vi "FunctionGenerator_New.vi"(11 "X Y Pairs":T1[](array[typedef]) {"Y" format="%_7f"; "X" format="%_7f"}) -> (3 "FUNCTION_GENERATOR":T2)   [LabVIEW 2019, in "Trajectory_Library.lvlib"]
doc: "Create a new Funtion Generator. Function Generators (Interpolating Tree Maps) are used to get values at points that are not defined by making a guess from points that are defined. This uses linear interpolation.\n\nInputs:\n - X Y Pairs -- (Optional) Array of pairs of X and Y values used to define this function generator. Additional X Y pairs can be added later. \n\nOutputs:\n - Function Generator -- Created data structure"
uses:
  Trajectory_Library.lvlib
  TypeDef/FUNCTION_GENERATOR.ctl
  X_Y_PAIR.ctl
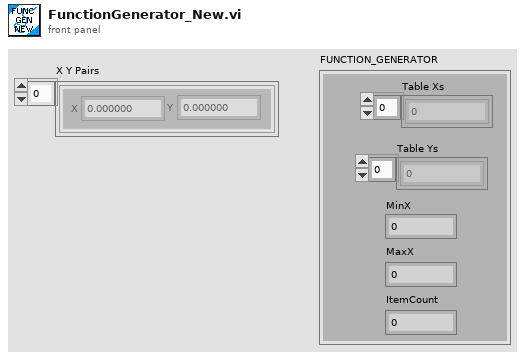
[diagram p1: front panel]
types:
  T1 = typedef "Trajectory_Library.lvlib/X_Y_PAIR.ctl" = cluster{"X":dbl, "Y":dbl}
  T2 = typedef "Trajectory_Library.lvlib/FUNCTION_GENERATOR.ctl" = cluster{"Table Xs":dbl[], "Table Ys":dbl[], "MinX":dbl, "MaxX":dbl, "ItemCount":i32}
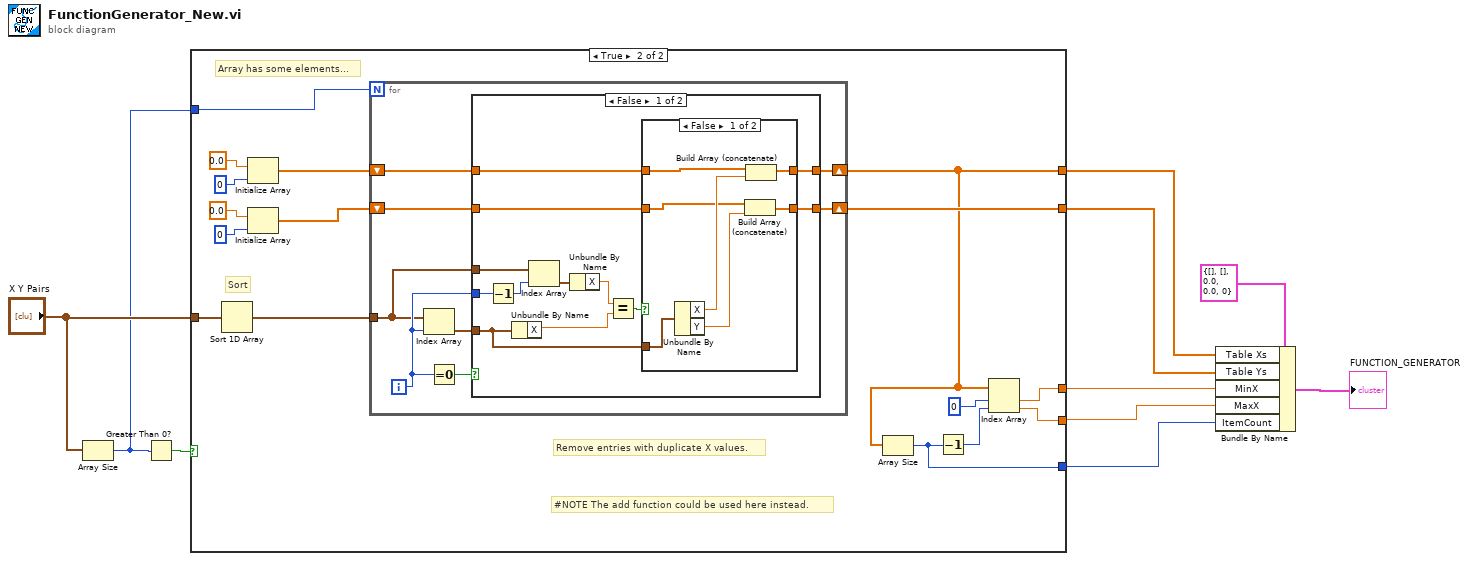
[diagram p0: block diagram]
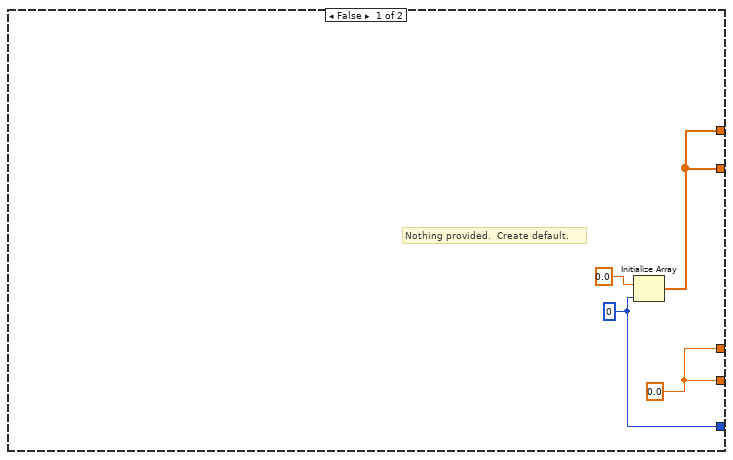
[diagram p2: hidden frame]
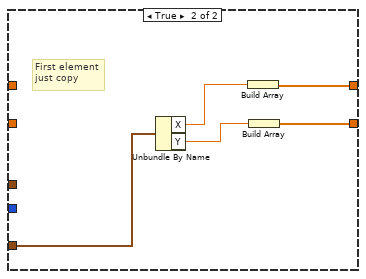
[diagram p4: hidden frame]
diagram:
  n1 = Array Size(array="X Y Pairs") -> (size(s)=w6:i32)
  n2 = Greater Than 0?(x=w6) -> (x > 0?=w8:bool)
  n3 = case shown="True" w8 {
    tunnel: "X Y Pairs" -> [_ w30]
    tunnel: w6 -> [_ w27]
    tunnel: [w13 w17] -> w5
    tunnel: [w13 w18] -> w4
    tunnel: [w12 w16] -> w3
    tunnel: [w12 w15] -> w2
    tunnel: [w11 w24] -> w1
    frame False {
      w12 = 0.0 ("X")
      w11 = 0 ("dimension size")
      # "Nothing provided.  Create default."
      n4 = Initialize Array(0.0 ("element"), w11) -> (w13:dbl[])
    }
    frame True {
      # "#NOTE The add function could be used here instead."
      # "Remove entries with duplicate X values."
      # "Sort"
      # "Array has some elements..."
      n5 = Sort 1D Array(array=w30) -> (sorted array=w26:T1[])
      n6 = Initialize Array(0.0, 0 ("dimension size")) -> (w20:dbl[])
      n7 = Initialize Array(0.0, 0 ("dimension size")) -> (w19:dbl[])
      n8 = for {
        N: w27 -> [_]
        tunnel: w26 -> [w35]
        shift-right: [w34] -> w17
        shift-left: w20 -> [w32]
        shift-right: [w33] -> w18
        shift-left: w19 -> [w31]
        i -> [w36]
        n9 = Index Array(array=w35, index=w36) -> (element=w37:T1)
        n10 = Equal To 0?(x=w36) -> (x = 0?=w38:bool)
        n11 = case shown="False" w38 {
          tunnel: w37 -> [w43 w64]
          tunnel: w36 -> [w49 _]
          tunnel: w35 -> [w48 _]
          tunnel: [w42 w63] -> w34
          tunnel: [w41 w62] -> w33
          tunnel: w32 -> [w40 _]
          tunnel: w31 -> [w39 _]
          frame False {
            n12 = Decrement(x=w49) -> (x-1=w50:i32)
            n13 = Unbundle By Name(w43) -> ("X"=w45:dbl)
            n14 = Index Array(array=w48, index=w50) -> (element=w47:T1)
            n15 = Unbundle By Name(w47) -> ("X"=w46:dbl)
            n16 = Equal?(x=w46, y=w45) -> (x = y?=w44:bool)
            n17 = case shown="False" w44 {
              tunnel: w43 -> [w55 _]
              tunnel: [w57 w59] -> w42
              tunnel: [w56 w58] -> w41
              tunnel: w40 -> [w52 w59]
              tunnel: w39 -> [w51 w58]
              frame False {
                n18 = Unbundle By Name(w55) -> ("X"=w54:dbl, "Y"=w53:dbl)
                n19 = Build Array (concatenate)(w51, w53) -> (w56:dbl[])
                n20 = Build Array (concatenate)(w52, w54) -> (w57:dbl[])
              }
              frame True {
                # "equal  x dont\ncopy element"
              }
            }
          }
          frame True {
            # "First element\njust copy"
            n21 = Unbundle By Name(w64) -> ("X"=w61:dbl, "Y"=w60:dbl)
            n22 = Build Array(w61) -> (w63:dbl[])
            n23 = Build Array(w60) -> (w62:dbl[])
          }
        }
      }
      n24 = Array Size(array=w17) -> (size(s)=w24:i32)
      n25 = Decrement(x=w24) -> (x-1=w28:i32)
      n26 = Index Array(array=w17, index #1=0 ("index"), index #2=w28) -> (element #1=w16:dbl, element #2=w15:dbl)
    }
  }
  n27 = Bundle By Name(cluster=T2 {"Table Xs"=[], "Table Ys"=[], "MinX"=0.0, "MaxX"=0.0, "ItemCount"=0} ("FUNCTION_GENERATOR"), "Table Xs"=w5, "Table Ys"=w4, "MinX"=w3, "MaxX"=w2, "ItemCount"=w1) -> (→"FUNCTION_GENERATOR":T2)
